vi "Check Event.vi"(9 "Distances Measure Array":dbl[](array[numeric]), 10 "Goal Frame (World)":cluster{"X":sgl, "Y":sgl, "Theta":dbl}, 11 "Robot Frame (World)":cluster{"X":sgl, "Y":sgl, "Theta":dbl}) -> (3 "Current Event":T2=enum."Go To Goal")   [LabVIEW 2016]
uses:
  RunningState.ctl
  Config for Running.ctl
panel:
  in  "Robot Config For Running in Meters":T1={"Dist. Stop (m)"=0.05, "Dist. Near Obs (m)"=0.2, "Dist. Dangerous (m)"=0.14}
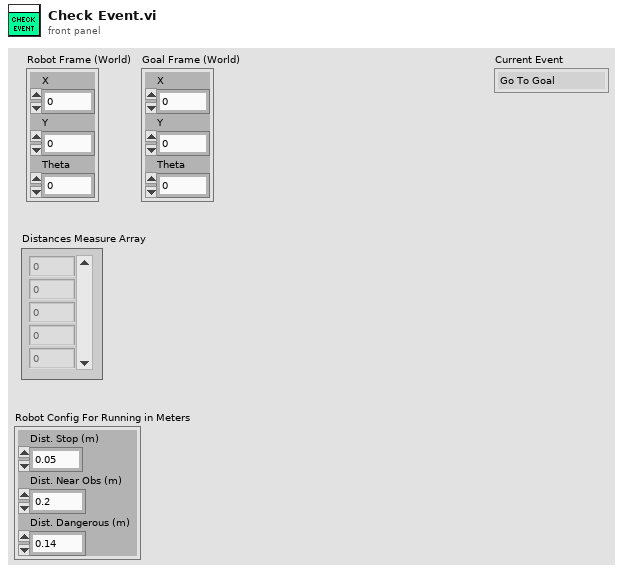
[diagram p1: front panel]
types:
  T1 = typedef "Config for Running.ctl" = cluster{"Dist. Stop (m)":sgl, "Dist. Near Obs (m)":dbl, "Dist. Dangerous (m)":dbl}
  T2 = typedef "RunningState.ctl" = enum16{"GTG and AO", "Go To Goal", "Wait", "Next Goal", "Avoid Obstacle", "Stop at Goal"}
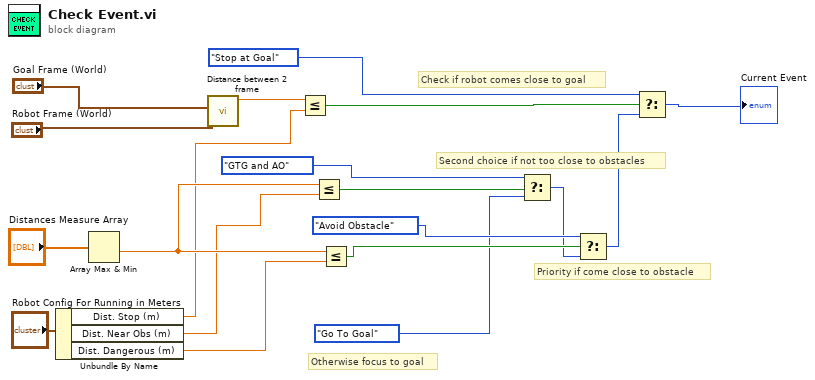
[diagram p0: block diagram]
diagram:
  # "Otherwise focus to goal"
  # "Second choice if not too close to obstacles"
  # "Priority if come close to obstacle"
  # "Check if robot comes close to goal"
  n1 = Unbundle By Name("Robot Config For Running in Meters") -> ("Dist. Stop (m)"=w4:sgl, "Dist. Near Obs (m)"=w3:dbl, "Dist. Dangerous (m)"=w2:dbl)
  n2 = Array Max & Min(array="Distances Measure Array") -> (min value=w13:dbl)  [unwired: 3 out]
  n3 = call "Distance between 2 frame.vi"("Goal Frame (World)"="Goal Frame (World)", "Robot Frame (World)"="Robot Frame (World)") -> ("sqrt(x)"=w17:sgl)  [unwired: 9 in]
  n4 = Less Or Equal?(x=w17, y=w4) -> (x <= y?=w16:bool)
  n5 = Less Or Equal?(x=w13, y=w3) -> (x <= y?=w12:bool)
  n6 = Less Or Equal?(x=w13, y=w2) -> (x <= y?=w10:bool)
  n7 = Select(t=RunningState."GTG and AO" ("Enum"), s=w12, f=RunningState."Go To Goal" ("Enum")) -> (s? t:f=w7:T2)
  n8 = Select(t=RunningState."Avoid Obstacle" ("Enum"), s=w10, f=w7) -> (s? t:f=w8:T2)
  n9 = Select(t=RunningState."Stop at Goal" ("Enum"), s=w16, f=w8) -> (s? t:f=→"Current Event":T2)
